vi "RTM - Add Channels.vi"(8 "error in (no error)":errorcluster, 11 "Node Ptr":u64 format="%.0x") -> (0 "error out":errorcluster)   [LabVIEW 2016, in "UDP-Custom-Device System Explorer.lvlib"]
uses:
  UDP-Custom-Device System Explorer.lvlib
  <vilib>/NI Veristand/Custom Device API/Custom Device Item Ref.ctl
  <vilib>/Utility/miscctls.llb/LVRowAndColumnUnsignedTypeDef.ctl
  <vilib>/NI Veristand/Custom Device API/Custom Device Channel Type.ctl
  <vilib>/NI VeriStand/Custom Device API/Custom Device API.lvlib
  <vilib>/NI VeriStand/Custom Device Tools/Custom Device Utility Library/Custom Device Utility Library.lvlib
  Property Accessors/Shared Packet Accessors.lvlib
panel:
  in  "Remove":bool
  in  "Selected Channels":i32[](listbox)
  in  "Add":bool
  in  "Available Channels":string[](tree)
  in  "OK":bool
  in  "Cancel":bool
  in  "Initial Selection":T1[](array[typedef]) format="%.0x"
  in  "Tag":string
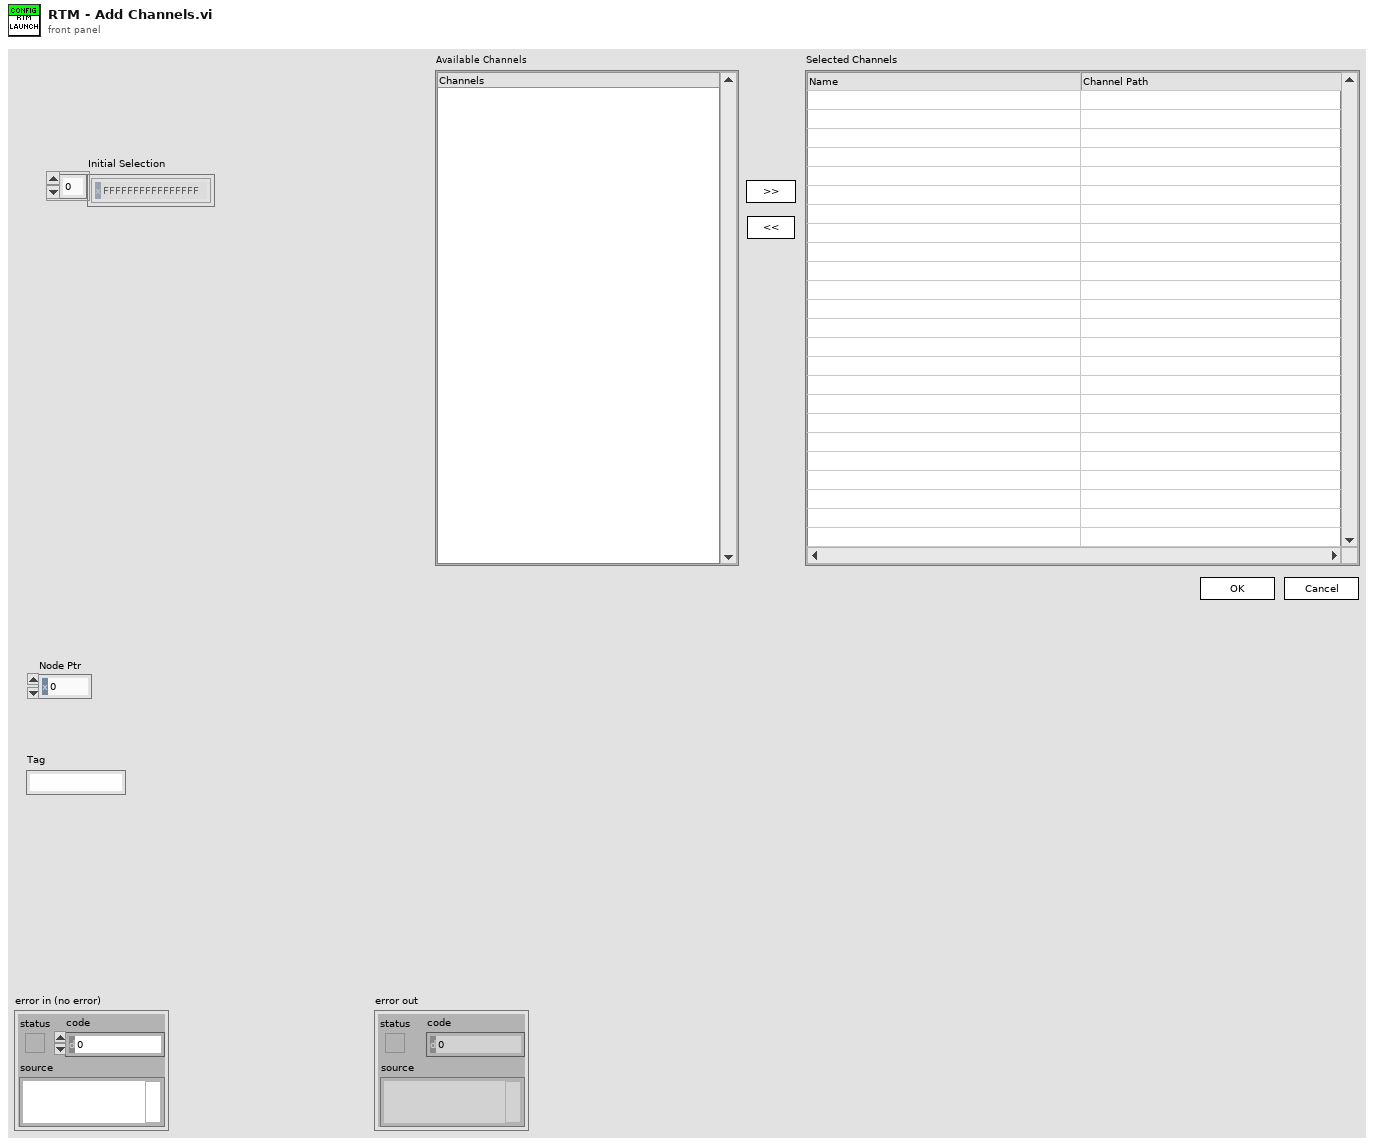
[diagram p1: front panel]
types:
  T1 = typedef "Custom Device API.lvlib/Custom Device Item Ref.ctl" = u64
  T2 = cluster{"Allow Section Selection (F)":bool, "Allow Multiple Selection (F)":bool}
  T3 = cluster{"Available Channels Label":string, "Selected Channels Label":string, "Mode":enum16{"Tx", "Rx"}}
  T4 = enum8{"Enabled", "Disabled", "Disabled and Grayed Out"}
  T5 = typedef "LVRowAndColumnUnsignedTypeDef.ctl" = cluster{"Row":u32, "Column":u32}
  T6 = typedef "Custom Device API.lvlib/Custom Device Channel Type.ctl" = enum16{"Input", "Output"}
  T7 = typedef "Custom Device API.lvlib/Custom Device Item Info.ctl" = cluster{"Name":string, "Is Channel":bool, "GUID":string, "Is Waveform":bool}
  T8 = typedef "Custom Device API.lvlib/Custom Device Channel.ctl" = cluster{"Type":T6, "Units":string, "Default Value":dbl, "Faultable":bool, "Scalable":bool}
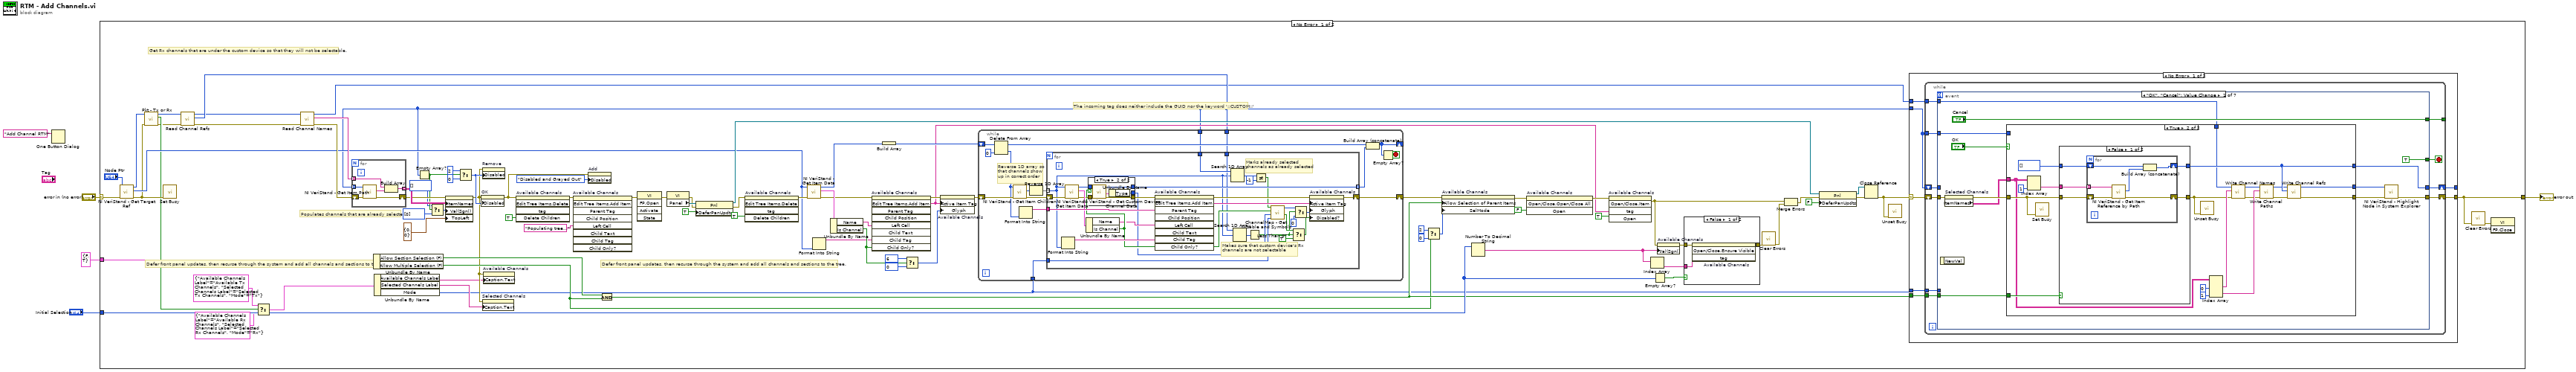
[diagram p0: block diagram]
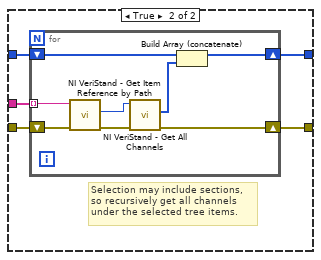
[diagram p4: hidden frame]
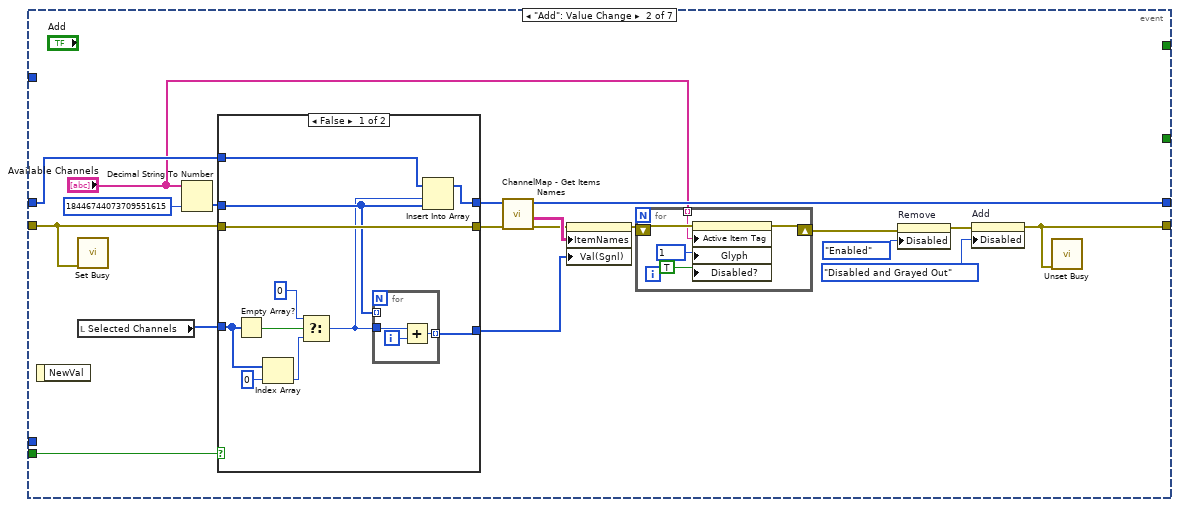
[diagram p5: hidden frame]
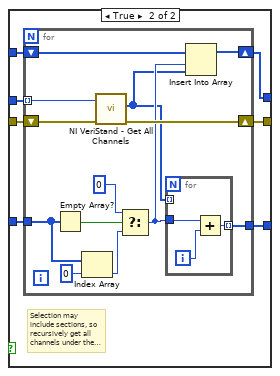
[diagram p6: hidden frame]
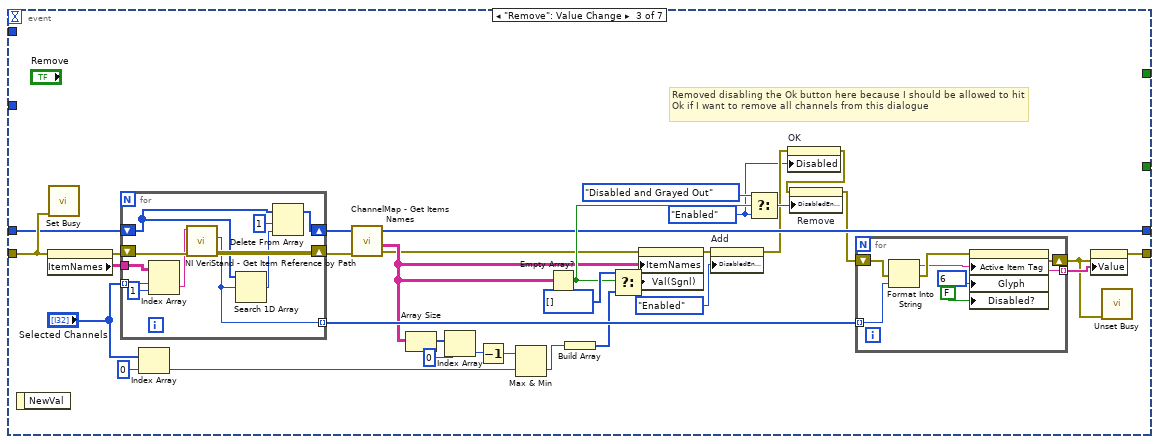
[diagram p7: hidden frame]
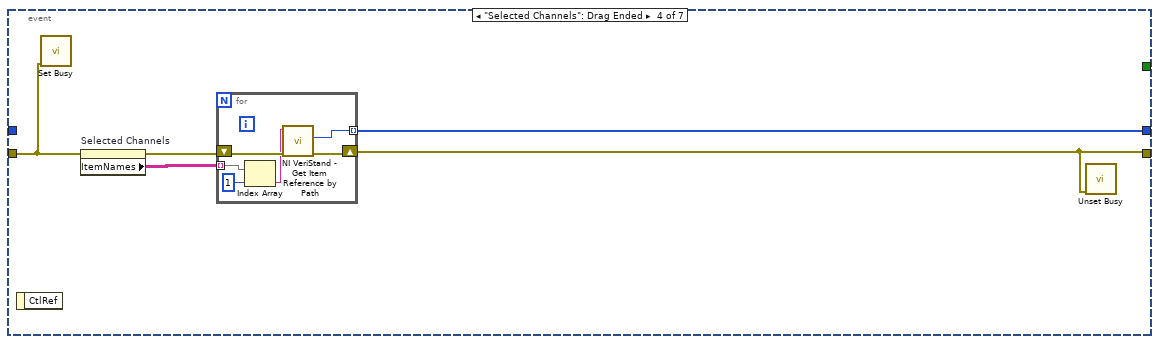
[diagram p8: hidden frame]
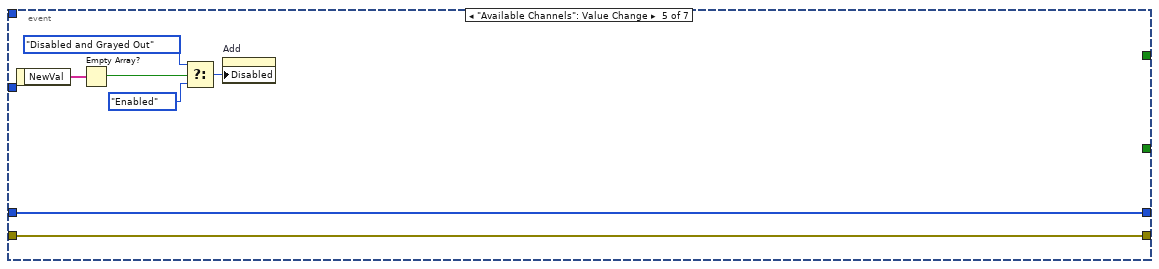
[diagram p9: hidden frame]
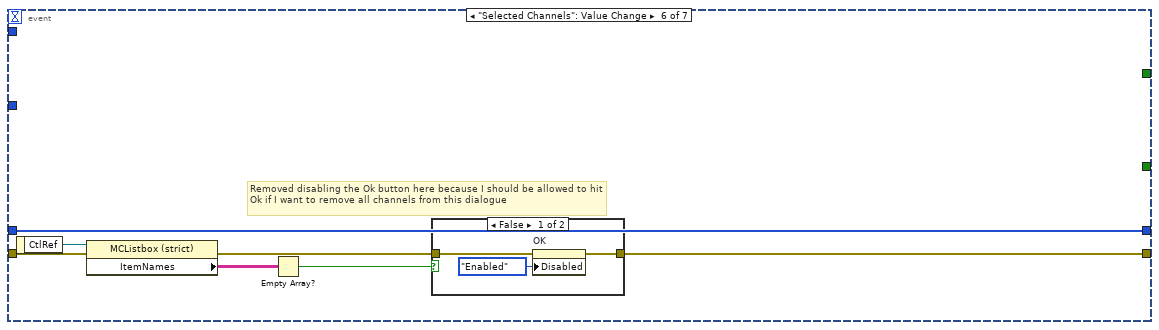
[diagram p10: hidden frame]
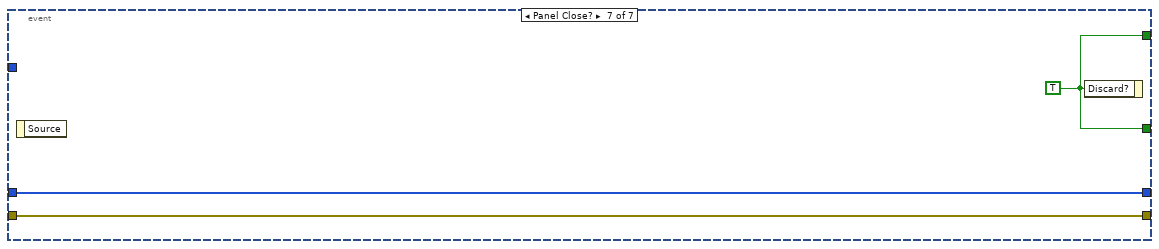
[diagram p12: hidden frame]
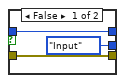
[diagram p14: hidden frame]
diagram:
  # "The incoming tag does neither include the GUID nor the keyword '::CUSTOM::'"
  n1 = One Button Dialog(message="Add Channel RTM") -> ()  [unwired: 1 in, 1 out]
  n2 = case shown="No Error" "error in (no error)" {
    selector: "error in (no error)" -> [w20 w376]
    tunnel: "Initial Selection" -> [w56 _]
    tunnel: [w74 w376] -> w2
    tunnel: T2 {"Allow Section Selection (F)"=FALSE, "Allow Multiple Selection (F)"=TRUE} ("Cluster") -> [w41 _]
    frame No Error {
      # "Defer front panel updates, then recurse through the system and add all channels and sections to the tree."
      # "Populates channels that are already selected"
      # "Get Rx channels that are under the custom device so that they will not be selectable."
      # "Defer front panel updates, then recurse through the system and add all channels and sections to the tree."
      n3 = call <vilib>:"NI VeriStand - Get Target Ref.vi"("error in"=w20, "Item Ref in"="Node Ptr") -> ("error out"=w16:errorcluster, "Target Ref"=w18:T1, "Item Ref out"=w17:T1)  [unwired: 6 in, 1 out]
      n4 = call "Pkt - Tx or Rx.vi"("error in (no error)"=w16, "Item Ref in"=w17) -> ("error out"=w10:errorcluster, "Tx?"=w13:bool, "Item Ref out"=w11:T1)  [unwired: 7 in]
      n5 = call <vilib>:"Set Busy.vi"("error in (no error)"=w16) -> ()  [unwired: 3 in, 8 out]
      n6 = call "Read Channel Refs.vi"("error in (no error)"=w10, "Node Ptr"=w11) -> ("error out"=w9:errorcluster, "Dependent Node Refs"=w8:T1[], "Node Ptr out"=w7:T1)  [unwired: 7 in]
      n7 = Select(t=T3 {"Available Channels Label"="Available Tx Channels", "Selected Channels Label"="Selected Tx Channels", "Mode"=enum."Tx"} ("Parameter"), s=w13, f=T3 {"Available Channels Label"="Available Rx Channels", "Selected Channels Label"="Selected Rx Channels", "Mode"=enum."Rx"} ("Parameter")) -> (s? t:f=w12:T3)
      n8 = call "Read Channel Names.vi"("error in (no error)"=w9, "Node Ptr"=w7) -> ("error out"=w22:errorcluster, "Channel Names"=w21:string[], "Node Ptr out"=w6:T1)  [unwired: 7 in]
      n9 = for {
        shift-right: [w94] -> w36
        shift-left: w22 -> [w96]
        tunnel: w8 -> [w95] mode=indexing
        tunnel: [w92] -> w37 mode=indexing
        tunnel: w21 -> [w91] mode=indexing
        n10 = call <vilib>:"NI VeriStand - Get Item Path.vi"("error in (no error)"=w96, "Item Ref in"=w95) -> ("error out"=w94:errorcluster, "Path"=w93:string)  [unwired: 8 out]
        n11 = Build Array(w91, w93) -> (w92:string[])
      }
      n12 = Unbundle By Name(w41) -> ("Allow Section Selection (F)"=w40:bool, "Allow Multiple Selection (F)"=w39:bool)
      n13 = Unbundle By Name(w12) -> ("Available Channels Label"=w25:string, "Selected Channels Label"=w24:string, "Mode"=w23:enum16{"Tx", "Rx"})
      n14 = Empty Array?(array=w8) -> (empty?=w30:bool)
      n15 = Select(t=i32[] [] ("Value (Signaling)"), s=w30, f=i32[] [0]) -> (s? t:f=w28:i32[])
      n16 = property on="Selected Channels" class="MCListbox (strict)"(error in=w36, "ItemNames"=w37, "Val(Sgnl)"=w28, "TopLeft"=T5 {"Row"=0, "Column"=0} ("Top Left Visible Cell")) -> (error out=w26:errorcluster)  [unwired: 1 in, 1 out]
      n17 = Select(t=u8 2, s=w30, f=u8 0) -> (s? t:f=w31:u8)
      n18 = property on="OK" class="Bool"(error in=w26, "Disabled"=w31) -> (error out=w33:errorcluster)  [unwired: 1 in, 1 out]
      n19 = property on="Remove" class="Bool"(error in=w26, "Disabled"=w31) -> ()  [unwired: 1 in, 2 out]
      n20 = property on="Selected Channels" class="MCListbox (strict)"(error in=w26, "Caption.Text"=w24) -> ()  [unwired: 1 in, 2 out]
      n21 = property on="Available Channels" class="Tree (strict)"(error in=w26, "Caption.Text"=w25) -> ()  [unwired: 1 in, 2 out]
      n22 = invoke on="Available Channels" class="Tree (strict)" method="Edit Tree Items.Delete"(error in=w33, "Delete Children"=TRUE ("Delete Children?")) -> (error out=w90:errorcluster)  [unwired: 3 in, 4 out]
      n23 = invoke on="Available Channels" class="Tree (strict)" method="Edit Tree Items.Add Item"(error in=w90, "Left Cell"="Populating tree..." ("Tag")) -> (error out=w87:errorcluster)  [unwired: 7 in, 8 out]
      n24 = property on="Add" class="Bool"(error in=w33, "Disabled"=T4."Disabled and Grayed Out") -> ()  [unwired: 1 in, 2 out]
      n25 = Compound Arithmetic op=AND(w40, w39) -> (w43:bool)
      n26 = invoke class="VI" method="FP.Open"(error in=w87) -> (error out=w85:errorcluster)  [unwired: 4 in, 4 out]
      n27 = property class="VI"(error in=w85) -> (error out=w83:errorcluster, "Panel"=w84:refnum<vi>)  [unwired: 1 in, 1 out]
      n28 = property class="Pnl"(reference=w84, error in=w83, "DeferPanUpdts"=TRUE ("Defer Panel Updates")) -> (reference out=w77:refnum<vi>, error out=w81:errorcluster)
      n29 = invoke on="Available Channels" class="Tree (strict)" method="Edit Tree Items.Delete"(error in=w81, "Delete Children"=TRUE ("Delete Children?")) -> (error out=w61:errorcluster)  [unwired: 3 in, 4 out]
      n30 = call <vilib>:"NI VeriStand - Get Item Data.vi"("error in (no error)"=w61, "Item Ref in"=w18) -> ("error out"=w64:errorcluster, "Item Info"=w66:T7, "Item Ref out"=w62:T1)  [unwired: 7 out]
      n31 = Format Into String(w18) -> (resulting string=w65:string)  [unwired: 3 in, 1 out]
      n32 = Unbundle By Name(w66) -> ("Name"=w67:string, "Is Channel"=w71:bool)
      n33 = invoke on="Available Channels" class="Tree (strict)" method="Edit Tree Items.Add Item"(error in=w64, "Left Cell"=w67, "Child Tag"=w65, "Child Only?"=w71) -> (error out=w68:errorcluster, "Edit Tree Items:Add Item"=w47:string)  [unwired: 5 in, 7 out]
      n34 = Build Array(w62) -> (w80:T1[])
      n35 = Select(t=6, s=w71, f=0) -> (s? t:f=w72:i32)
      n36 = property on="Available Channels" class="Tree (strict)"(error in=w68, "Active Item Tag"=w47, "Glyph"=w72) -> (error out=w63:errorcluster)  [unwired: 1 in, 1 out]
      n37 = while {
        shift-right: [w328] -> w79
        shift-left: w63 -> [w334]
        shift-right: [w333] -> _
        shift-left: w80 -> [w337]
        tunnel: w8 -> [w325]
        tunnel: w23 -> [w324]
        tunnel: w8 -> [w323]
        stop <- w332 stop-if-true
        # "Reverse 1D array so that channels show up in correct order"
        n38 = Delete From Array(array=w337, index=0) -> (deleted portion=w327:T1, array with subset deleted=w335:T1[])  [unwired: 1 in]
        n39 = call <vilib>:"NI VeriStand - Get Item Children.vi"("error in (no error)"=w334, "Item Ref in"=w327) -> ("error out"=w331:errorcluster, "Child Refs"=w330:T1[])  [unwired: 8 out]
        n40 = Format Into String(w327) -> (resulting string=w326:string)  [unwired: 3 in, 1 out]
        n41 = Reverse 1D Array(array=w330) -> (reversed array=w322:T1[])
        n42 = for {
          shift-right: [w360] -> w328
          shift-left: w331 -> [w365]
          tunnel: w322 -> [w347] mode=indexing
          tunnel: [w357] -> w329 mode=indexing
          tunnel: w326 -> [w366]
          tunnel: w325 -> [w359]
          tunnel: w324 -> [w351]
          tunnel: w323 -> [w348]
          # "Marks already selected channels as already selected"
          # "Makes sure that custom device's Rx channels are not selectable"
          n43 = Format Into String(w347) -> (resulting string=w364:string)  [unwired: 3 in, 1 out]
          n44 = call <vilib>:"NI VeriStand - Get Item Data.vi"("error in (no error)"=w365, "Item Ref in"=w347) -> ("error out"=w356:errorcluster, "Item Info"=w363:T7, "Item Ref out"=w358:T1)  [unwired: 7 out]
          n45 = Unbundle By Name(w363) -> ("Name"=w349:string, "Is Channel"=w350:bool)
          n46 = case shown="True" w350 {
            tunnel: w358 -> [w369 w375]
            tunnel: [w369 w374] -> w357
            tunnel: w356 -> [w368 w373]
            tunnel: [w368 w372] -> w355
            tunnel: [Custom_Device_Channel_Type."Input" ("Type") w370] -> w345
            frame False {
            }
            frame True {
              n47 = call <vilib>:"NI VeriStand - Get Custom Device Channel Data.vi"("error in (no error)"=w373, "Channel Ref in"=w375) -> ("error out"=w372:errorcluster, "Channel"=w371:T8, "Channel Ref out"=w374:T1)  [unwired: 4 in, 3 out]
              n48 = Unbundle By Name(w371) -> ("Type"=w370:T6)
            }
          }
          n49 = invoke on="Available Channels" class="Tree (strict)" method="Edit Tree Items.Add Item"(error in=w355, "Parent Tag"=w366, "Left Cell"=w349, "Child Tag"=w364, "Child Only?"=w350) -> (error out=w362:errorcluster, "Edit Tree Items:Add Item"=w361:string)  [unwired: 4 in, 7 out]
          n50 = Search 1D Array(1D array=w359, element=w347) -> (index of element=w354:i32)  [unwired: 1 in]
          n51 = Search 1D Array(1D array=w348, element=w347) -> (index of element=w346:i32)  [unwired: 1 in]
          n52 = Less Than 0?(x=w346) -> (x < 0?=w339:bool)
          n53 = Not Equal?(x=w354, y=-1) -> (x != y?=w352:bool)
          n54 = call "ChannelMap - Get Disable and Symbols.vi"("Mode"=w351, "Channel Type"=w345, "Is Channel?"=w350, "Is Selected?"=w352) -> ("Disabled?"=w344:bool, "Symbole"=w341:i32)  [unwired: 6 in]
          n55 = Select(t=w344, s=w339, f=TRUE) -> (s? t:f=w343:bool)
          n56 = Select(t=w341, s=w339, f=0) -> (s? t:f=w340:i32)
          n57 = property on="Available Channels" class="Tree (strict)"(error in=w362, "Active Item Tag"=w361, "Glyph"=w340, "Disabled?"=w343) -> (error out=w360:errorcluster)  [unwired: 1 in, 1 out]
        }
        n58 = Build Array (concatenate)(w335, w329) -> (w333:T1[])
        n59 = Empty Array?(array=w333) -> (empty?=w332:bool)
      }
      n60 = Select(t=2 ("Selection Mode"), s=w39, f=0 ("Selection Mode")) -> (s? t:f=w44:i32)
      n61 = property on="Available Channels" class="Tree (strict)"(error in=w79, "Allow Selection of Parent Items"=w43, "SelMode"=w44) -> (error out=w52:errorcluster)  [unwired: 1 in, 1 out]
      n62 = Number To Decimal String(number=w56) -> (decimal integer string=w54:string[])  [unwired: 1 out]
      n63 = invoke on="Available Channels" class="Tree (strict)" method="Open/Close.Open/Close All"(error in=w52, "Open"=FALSE ("Open?")) -> (error out=w50:errorcluster)  [unwired: 2 in, 3 out]
      n64 = invoke on="Available Channels" class="Tree (strict)" method="Open/Close.Item"(error in=w50, "tag"=w47, "Open"=TRUE ("Open?")) -> (error out=w48:errorcluster)  [unwired: 2 in, 4 out]
      n65 = Index Array(array=w54) -> (element=w53:string)  [unwired: 1 in]
      n66 = Empty Array?(array=w56) -> (empty?=w55:bool)
      n67 = property on="Available Channels" class="Tree (strict)"(error in=w48, "Val(Sgnl)"=w54) -> (error out=w58:errorcluster)  [unwired: 1 in, 1 out]
      n68 = case shown="False" w55 {
        tunnel: w58 -> [w99 w100]
        tunnel: [w98 w100] -> w57
        tunnel: w53 -> [w97 _]
        frame False {
          n69 = invoke on="Available Channels" class="Tree (strict)" method="Open/Close.Ensure Visible"(error in=w99, "tag"=w97) -> (error out=w98:errorcluster)  [unwired: 2 in, 3 out]
        }
        frame True {
        }
      }
      n70 = call <vilib>:"Clear Errors.vi"("error in (no error)"=w57) -> ("error out"=w60:errorcluster)  [unwired: 1 in, 5 out]
      n71 = Merge Errors(w48, w60) -> (w59:errorcluster)
      n72 = property class="Pnl"(reference=w77, error in=w59, "DeferPanUpdts"=FALSE ("Defer Panel Updates")) -> (reference out=w75:refnum<vi>, error out=w76:errorcluster)
      n73 = Close Reference(reference=w75, error in (no error)=w76) -> (error out=w42:errorcluster)
      n74 = call <vilib>:"Unset Busy.vi"("error in (no error)"=w42) -> ()  [unwired: 1 in, 10 out]
      n75 = case shown="No Error" w42 {
        selector: w42 -> [w107 w321]
        tunnel: [w106 w321] -> w74
        tunnel: [w105 w320] -> _
        tunnel: w43 -> [w104 _]
        tunnel: w8 -> [w103 w320]
        tunnel: w23 -> [w102 _]
        tunnel: w6 -> [w101 _]
        frame No Error {
          n76 = while {
            shift-right: [w116] -> w106
            shift-left: w107 -> [w117]
            tunnel: [w115] -> _
            tunnel: w104 -> [w113]
            shift-right: [w110] -> w105
            shift-left: w103 -> [w112]
            tunnel: w103 -> [w111]
            tunnel: w102 -> [w109]
            tunnel: w101 -> [w108]
            stop <- w114 stop-if-true
            n77 = event shown="[0] \"OK\", \"Cancel\": Value Change" {
              selector: _ -> [_ _ _ _ _ _ _]
              dyn-events: _ -> [_ _ _ _ _ _ _]
              timeout: _ -> [_ _ _ _ _ _ _]
              tunnel: w117 -> [w126 w193 w269 w292 w305 w310 w319]
              tunnel: [w122 w177 w242 w289 w305 w307 w319] -> w116
              tunnel: ["Cancel" _ _ _ _ _ w318] -> w115
              tunnel: [TRUE ("Discard?") _ _ _ _ _ w318] -> w114
              tunnel: [w118 w189 w248 w288 w302 w312 w317] -> w110
              tunnel: w113 -> [w128 w192 _ _ _ _ _]
              tunnel: w112 -> [_ w191 w266 _ w302 w312 w317]
              tunnel: w111 -> [w124 _ _ _ _ _ _]
              tunnel: w109 -> [_ _ _ _ _ _ _]
              tunnel: w108 -> [w121 _ _ _ _ _ _]
              event "OK", "Cancel": Value Change {
                n78 = event-data() -> ()  [unwired: 2 out]
                n79 = property on="Selected Channels" class="MCListbox (strict)"(error in=w126) -> (error out=w125:errorcluster, "ItemNames"=w123:string[][])  [unwired: 1 in, 1 out]
                n80 = case shown="True" "OK" {
                  tunnel: w123 -> [_ w145]
                  tunnel: w128 -> [_ w152]
                  tunnel: w125 -> [w133 w150]
                  tunnel: [w132 w144] -> w118
                  tunnel: [w133 w143] -> w119
                  tunnel: w124 -> [w132 _]
                  tunnel: w121 -> [w131 w141]
                  tunnel: [w131 w142] -> w120
                  frame False {
                  }
                  frame True {
                    n81 = Index Array(array=w145, index (col)=1 ("disabled index (col)")) -> (element=w148:string[])  [unwired: 1 in]
                    n82 = call <vilib>:"Set Busy.vi"("error in (no error)"=w150) -> ()  [unwired: 3 in, 8 out]
                    n83 = case shown="False" w152 {
                      tunnel: w150 -> [w157 w168]
                      tunnel: [w153 w166] -> w144
                      tunnel: [w156 w165] -> w139
                      tunnel: T1[] [] ("Channel Refs") -> [w154 w167]
                      tunnel: w148 -> [w155 w164]
                      frame False {
                        n84 = for {
                          tunnel: w155 -> [w161] mode=indexing
                          shift-right: [w158] -> w153
                          shift-left: w154 -> [w159]
                          shift-right: [w162] -> w156
                          shift-left: w157 -> [w163]
                          n85 = call <vilib>:"NI VeriStand - Get Item Reference by Path.vi"("error in (no error)"=w163, "Item Path in"=w161) -> ("error out"=w162:errorcluster, "Item Ref"=w160:T1)  [unwired: 6 in, 2 out]
                          n86 = Build Array (concatenate)(w159, w160) -> (w158:T1[])
                        }
                      }
                      frame True {
                        # "Selection may include sections, so recursively get all channels under the selected tree items."
                        n87 = for {
                          shift-right: [w174] -> w166
                          shift-left: w167 -> [w175]
                          shift-right: [w176] -> w165
                          shift-left: w168 -> [w171]
                          tunnel: w164 -> [w172] mode=indexing
                          n88 = call <vilib>:"NI VeriStand - Get Item Reference by Path.vi"("error in (no error)"=w171, "Item Path in"=w172) -> ("error out"=w170:errorcluster, "Item Ref"=w169:T1)  [unwired: 6 in, 2 out]
                          n89 = call <vilib>:"NI VeriStand - Get All Channels.vi"("error in"=w170, "Section Ref in"=w169) -> ("error out"=w176:errorcluster, "Channel Refs"=w173:T1[])  [unwired: 8 out]
                          n90 = Build Array (concatenate)(w175, w173) -> (w174:T1[])
                        }
                      }
                    }
                    n91 = call <vilib>:"Unset Busy.vi"("error in (no error)"=w139) -> ()  [unwired: 1 in, 10 out]
                    n92 = Index Array(array=w145, index (col) #1=0 ("disabled index (col)"), index (col) #2=1 ("index (col)")) -> (element #1=w140:string[], element #2=w137:string[])  [unwired: 2 in]
                    n93 = call "Write Channel Names.vi"("error in (no error)"=w139, "Channel Names"=w140, "Node Ptr"=w141) -> ("error out"=w136:errorcluster, "Node Ptr out"=w138:T1)  [unwired: 7 in]
                    n94 = call "Write Channel Paths.vi"("error in (no error)"=w136, "Channel Paths"=w137, "Node Ptr"=w138) -> ("error out"=w135:errorcluster, "Node Ptr out"=w134:T1)  [unwired: 7 in]
                    n95 = call "Write Channel Refs.vi"("error in (no error)"=w135, "Dependent Node Refs"=w144, "Node Ptr"=w134) -> ("error out"=w143:errorcluster, "Node Ptr out"=w142:T1)  [unwired: 7 in]
                  }
                }
                n96 = call <vilib>:"NI VeriStand - Highlight Node in System Explorer.vi"("error in (no error)"=w119, "Item Ref in"=w120) -> ("error out"=w122:errorcluster)  [unwired: 8 in, 1 out]
              }
              event "Add": Value Change {
                n97 = event-data() -> ()  [unwired: 2 out]
                n98 = call <vilib>:"Set Busy.vi"("error in (no error)"=w193) -> ()  [unwired: 3 in, 8 out]
                n99 = local read "Selected Channels"() -> (w181:i32[])
                n100 = Decimal String To Number(string="Available Channels", default (0L)=T1 18446744073709551615 ("Device Item Ref")) -> (number=w195:u64[])  [unwired: 2 out]
                n101 = case shown="False" w192 {
                  tunnel: w193 -> [w211 w221]
                  tunnel: [w208 w220] -> w190
                  tunnel: w195 -> [w203 w219]
                  tunnel: [w211 w218] -> w188
                  tunnel: w191 -> [w209 w217]
                  tunnel: w181 -> [w207 w216]
                  tunnel: [w201 w215] -> w180
                  frame False {
                    n102 = Empty Array?(array=w207) -> (empty?=w210:bool)
                    n103 = Index Array(array=w207, index=0) -> (element=w205:i32)
                    n104 = Select(t=0, s=w210, f=w205) -> (s? t:f=w202:i32)
                    n105 = for {
                      tunnel: w203 -> [_] mode=indexing
                      tunnel: w202 -> [w214]
                      tunnel: [w212] -> w201 mode=indexing
                      i -> [w213]
                      n106 = Add(x=w214, y=w213) -> (x+y=w212:i32)
                    }
                    n107 = Insert Into Array(array=w209, index=w202, new element=w203) -> (w208:T1[])
                  }
                  frame True {
                    # "Selection may include sections, so recursively get all channels under the selected tree items."
                    n108 = for {
                      shift-right: [w226] -> w220
                      shift-left: w217 -> [w225]
                      shift-right: [w233] -> w218
                      shift-left: w221 -> [w234]
                      tunnel: w219 -> [w232] mode=indexing
                      tunnel: w216 -> [w227]
                      tunnel: [w224] -> w215
                      n109 = Empty Array?(array=w227) -> (empty?=w228:bool)
                      n110 = Index Array(array=w227, index=0) -> (element=w230:i32)
                      n111 = call <vilib>:"NI VeriStand - Get All Channels.vi"("error in"=w234, "Section Ref in"=w232) -> ("error out"=w233:errorcluster, "Channel Refs"=w222:T1[])  [unwired: 8 out]
                      n112 = Select(t=0, s=w228, f=w230) -> (s? t:f=w223:i32)
                      n113 = for {
                        tunnel: w223 -> [w237]
                        tunnel: [w235] -> w224 mode=indexing
                        tunnel: w222 -> [_] mode=indexing
                        i -> [w236]
                        n114 = Add(x=w237, y=w236) -> (x+y=w235:i32)
                      }
                      n115 = Insert Into Array(array=w225, index=w223, new element=w222) -> (w226:T1[])
                    }
                  }
                }
                n116 = call "ChannelMap - Get Items Names.vi"("error IO 2"=w188, "TCP Channel Refs In"=w190) -> ("error IO"=w183:errorcluster, "Items Names"=w184:string[][], "TCP Channel Refs Out"=w189:T1[])  [unwired: 7 in]
                n117 = property on="Selected Channels" class="MCListbox (strict)"(error in=w183, "ItemNames"=w184, "Val(Sgnl)"=w180) -> (error out=w187:errorcluster)  [unwired: 1 in, 1 out]
                n118 = for {
                  shift-right: [w199] -> w179
                  shift-left: w187 -> [w200]
                  tunnel: "Available Channels" -> [w197] mode=indexing
                  n119 = property on="Available Channels" class="Tree (strict)"(error in=w200, "Active Item Tag"=w197, "Glyph"=1, "Disabled?"=TRUE ("Active Item:Disabled?")) -> (error out=w199:errorcluster)  [unwired: 1 in, 1 out]
                }
                n120 = property on="Remove" class="Bool"(error in=w179, "Disabled"=T4."Enabled") -> (error out=w178:errorcluster)  [unwired: 1 in, 1 out]
                n121 = property on="Add" class="Bool"(error in=w178, "Disabled"=T4."Disabled and Grayed Out") -> (error out=w177:errorcluster)  [unwired: 1 in, 1 out]
                n122 = call <vilib>:"Unset Busy.vi"("error in (no error)"=w177) -> ()  [unwired: 1 in, 10 out]
              }
              event "Remove": Value Change {
                w239 = T4."Enabled" ("Disabled")
                # "Removed disabling the Ok button here because I should be allowed to hit Ok if I want to remove all channels from this dialogue"
                n123 = event-data() -> ()  [unwired: 2 out]
                n124 = property on="Selected Channels" class="MCListbox (strict)"(error in=w269) -> (error out=w268:errorcluster, "ItemNames"=w267:string[][])  [unwired: 1 in, 1 out]
                n125 = call <vilib>:"Set Busy.vi"("error in (no error)"=w269) -> ()  [unwired: 3 in, 8 out]
                n126 = for {
                  tunnel: w267 -> [w278]
                  tunnel: "Selected Channels" -> [w279] mode=indexing
                  shift-right: [w277] -> w250
                  shift-left: w268 -> [w280]
                  shift-right: [w275] -> w247
                  shift-left: w266 -> [w276]
                  tunnel: [w272] -> w265 mode=indexing
                  n127 = Index Array(array=w278, index (row)=w279, index (col)=1 ("disabled index (col)")) -> (element=w270:string)
                  n128 = call <vilib>:"NI VeriStand - Get Item Reference by Path.vi"("error in (no error)"=w280, "Item Path in"=w270) -> ("error out"=w277:errorcluster, "Item Ref"=w272:T1)  [unwired: 6 in, 2 out]
                  n129 = Search 1D Array(1D array=w276, element=w272) -> (index of element=w273:i32)  [unwired: 1 in]
                  n130 = Delete From Array(array=w276, length=1, index=w273) -> (array with subset deleted=w275:T1[])  [unwired: 1 out]
                }
                n131 = Index Array(array="Selected Channels", index=0) -> (element=w253:i32)
                n132 = call "ChannelMap - Get Items Names.vi"("error IO 2"=w250, "TCP Channel Refs In"=w247) -> ("error IO"=w246:errorcluster, "Items Names"=w249:string[][], "TCP Channel Refs Out"=w248:T1[])  [unwired: 7 in]
                n133 = Array Size(array=w249) -> (size(s)=w257:i32[])
                n134 = Index Array(array=w257, index=0) -> (element=w255:i32)
                n135 = Decrement(x=w255) -> (x-1=w254:i32)
                n136 = Max & Min(x=w254, y=w253) -> (min(x,y)=w252:i32)  [unwired: 1 out]
                n137 = Empty Array?(array=w249) -> (empty?=w262:bool)
                n138 = Build Array(w252) -> (w259:i32[])
                n139 = Select(t=i32[] [] ("Selected TCP Channels"), s=w262, f=w259) -> (s? t:f=w263:i32[])
                n140 = property on="Selected Channels" class="MCListbox (strict)"(error in=w246, "ItemNames"=w249, "Val(Sgnl)"=w263) -> ()  [unwired: 1 in, 2 out]
                n141 = property on="Add" class="Bool"(error in=w246, "DisabledEnum"=T4."Enabled" ("Disabled")) -> (error out=w245:errorcluster)  [unwired: 1 in, 1 out]
                n142 = Select(t=T4."Disabled and Grayed Out" ("Disabled"), s=w262, f=w239) -> (s? t:f=w261:T4)
                n143 = property on="OK" class="Bool"(error in=w245, "Disabled"=w239) -> (error out=w244:errorcluster)  [unwired: 1 in, 1 out]
                n144 = property on="Remove" class="Bool"(error in=w244, "DisabledEnum"=w261) -> (error out=w243:errorcluster)  [unwired: 1 in, 1 out]
                n145 = for {
                  shift-right: [w285] -> w241
                  shift-left: w243 -> [w283]
                  tunnel: w265 -> [w284] mode=indexing
                  tunnel: [w281] -> w251 mode=indexing
                  n146 = Format Into String(error in=w283, w284) -> (resulting string=w281:string, error out=w282:errorcluster)  [unwired: 2 in]
                  n147 = property on="Available Channels" class="Tree (strict)"(error in=w282, "Active Item Tag"=w281, "Glyph"=6, "Disabled?"=FALSE ("Active Item:Disabled?")) -> (error out=w285:errorcluster)  [unwired: 1 in, 1 out]
                }
                n148 = property on="Available Channels" class="Tree (strict)"(error in=w241, "Value"=w251) -> (error out=w242:errorcluster)  [unwired: 1 in, 1 out]
                n149 = call <vilib>:"Unset Busy.vi"("error in (no error)"=w241) -> ()  [unwired: 1 in, 10 out]
              }
              event "Selected Channels": Drag Ended {
                n150 = event-data() -> ()  [unwired: 2 out]
                n151 = call <vilib>:"Set Busy.vi"("error in (no error)"=w292) -> ()  [unwired: 3 in, 8 out]
                n152 = property on="Selected Channels" class="MCListbox (strict)"(error in=w292) -> (error out=w291:errorcluster, "ItemNames"=w290:string[][])  [unwired: 1 in, 1 out]
                n153 = for {
                  tunnel: w290 -> [w297] mode=indexing
                  shift-right: [w296] -> w289
                  shift-left: w291 -> [w298]
                  tunnel: [w295] -> w288 mode=indexing
                  n154 = Index Array(array=w297, index=1 ("disabled index (col)")) -> (element=w294:string)
                  n155 = call <vilib>:"NI VeriStand - Get Item Reference by Path.vi"("error in (no error)"=w298, "Item Path in"=w294) -> ("error out"=w296:errorcluster, "Item Ref"=w295:T1)  [unwired: 6 in, 2 out]
                }
                n156 = call <vilib>:"Unset Busy.vi"("error in (no error)"=w289) -> ()  [unwired: 1 in, 10 out]
              }
              event "Available Channels": Value Change {
                n157 = event-data() -> ("NewVal"=w304:string[])  [unwired: 1 out]
                n158 = Empty Array?(array=w304) -> (empty?=w301:bool)
                n159 = Select(t=T4."Disabled and Grayed Out" ("Disabled"), s=w301, f=T4."Enabled" ("Disabled")) -> (s? t:f=w303:T4)
                n160 = property on="Add" class="Bool"("Disabled"=w303) -> ()  [unwired: 2 in, 2 out]
              }
              event "Selected Channels": Value Change {
                # "Removed disabling the Ok button here because I should be allowed to hit Ok if I want to remove all channels from this dialogue"
                n161 = event-data() -> ("CtlRef"=w311:refnum<vi>)  [unwired: 1 out]
                n162 = property class="MCListbox (strict)"(reference=w311, error in=w310) -> (error out=w308:errorcluster, "ItemNames"=w309:string[][])  [unwired: 1 out]
                n163 = Empty Array?(array=w309) -> (empty?=w306:bool)
                n164 = case shown="False" w306 {
                  tunnel: w308 -> [w315 w316]
                  tunnel: [w314 w316] -> w307
                  frame False {
                    n165 = property on="OK" class="Bool"(error in=w315, "Disabled"=T4."Enabled") -> (error out=w314:errorcluster)  [unwired: 1 in, 1 out]
                  }
                  frame True {
                  }
                }
              }
              event Panel Close? {
                w318 = TRUE ("Discard?")
                n166 = event-data() -> ()  [unwired: 2 out]
                n167 = event-data("Discard?"=w318) -> ()  [unwired: 1 in, 1 out]
              }
            }
          }
        }
        frame Error {
        }
      }
      n168 = call <vilib>:"Clear Errors.vi"("error in (no error)"=w74) -> ("error out"=w73:errorcluster)  [unwired: 1 in, 5 out]
      n169 = invoke class="VI" method="FP.Close"(error in=w73) -> ()  [unwired: 2 in, 3 out]
    }
    frame Error {
    }
  }
  "error out" <- w2
